vi "Get Available Operating Modes.vi"(8 "error in (no error)":errorcluster, 11 "VISA resource name":refnum<visa-resource-name>) -> (0 "error out":errorcluster, 2 "Operating Modes":i32[](array[ring]) items=["Weighing", "Parts Counting", "Deviations", "Dosing", "Formulas", "Animals Weighing", "Density", "Density of Solid Bodies", "Density of Liquids", "Peak Hold", "Totalizing", "Checkweighin", "Statistics", "Pipettes Calibration", "Differential Weighing", "Statistical Quality Control (SQC)", "Product Inspection", "Weight Control (Tableting)", "Drying", "Comparator", "Weighbridge"], 3 "VISA resource name out":refnum<visa-resource-name>)   [LabVIEW 2017, in "RadWag balances and scales.lvlib"]
doc: "Reads operating modes which are suported in connected balance.\nUsage of this VI is highly recommended before running VI \"Set Operating Mode\".\nTo see recommended usage of VI connected with seting operating mode open Examples ->RadWag Counting Pieces."
uses:
  <instrlib>/Prev/RadWag Continuous Read Folder/RadWag balances and scales.lvlib
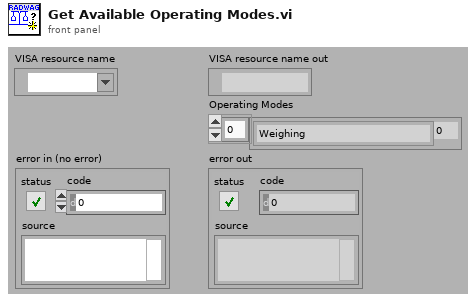
[diagram p1: front panel]
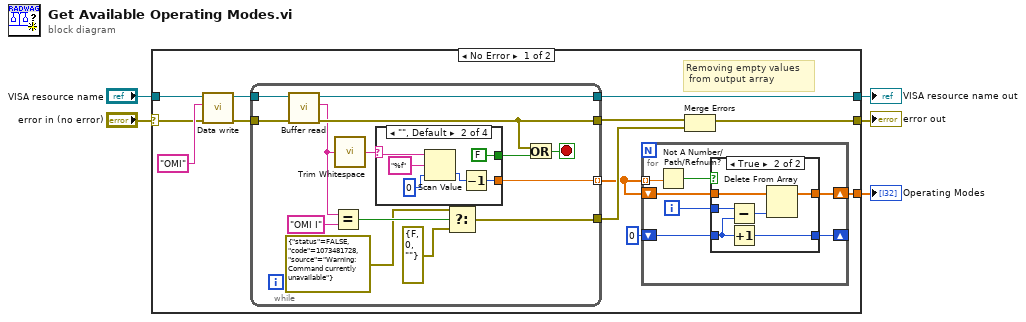
[diagram p0: block diagram]
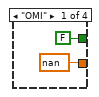
[diagram p3: hidden frame]
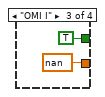
[diagram p4: hidden frame]
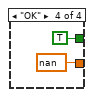
[diagram p5: hidden frame]
diagram:
  n1 = case shown="No Error" "error in (no error)" {
    selector: "error in (no error)" -> [w10 w59]
    tunnel: "VISA resource name" -> [w17 w60]
    tunnel: [w7 w59] -> w3
    tunnel: [w12 w60] -> w2
    tunnel: [w11 _] -> w1
    frame No Error {
      # "Removing empty values\n from output array"
      n2 = call <instrlib>:"Data write.vi"("error in (no error)"=w10, "ID"="OMI", "VISA resource name"=w17) -> ("error out"=w15:errorcluster, "VISA resource name out"=w16:refnum<visa-resource-name>)  [unwired: 7 in]
      n3 = while {
        tunnel: w16 -> [w46]
        tunnel: w15 -> [w45]
        tunnel: [w44] -> w12
        tunnel: [w42] -> w8
        tunnel: [w33] -> w6 mode=indexing
        tunnel: [w36] -> w9
        stop <- w40 stop-if-true
        n4 = call <instrlib>:"Buffer read.vi"("error in (no error)"=w45, "VISA resource name"=w46) -> ("error out"=w42:errorcluster, "Received String"=w35:string, "VISA resource name out"=w44:refnum<visa-resource-name>)  [unwired: 7 in]
        n5 = Equal?(x=w35, y="OMI I") -> (x = y?=w39:bool)
        n6 = call <vilib>:"Trim Whitespace.vi"("string"=w35) -> ("trimmed string"=w34:string)  [unwired: 1 in]
        n7 = case shown="\"\", Default" w34 {
          selector: w34 -> [_ w53 _ _]
          tunnel: [FALSE FALSE TRUE TRUE] -> w41
          tunnel: [nan w49 nan nan] -> w33
          frame "OMI" {
          }
          frame "", Default {
            n8 = Scan Value(string=w53, format string="%f", default (0 dbl)=0) -> (value=w50:i32)  [unwired: 1 out]
            n9 = Decrement(x=w50) -> (x-1=w49:i32)
          }
          frame "OMI I" {
          }
          frame "OK" {
          }
        }
        n10 = Select(t=errorcluster {"status"=FALSE, "code"=1073481728, "source"="Warning: Command currently unavailable"}, s=w39, f=errorcluster {"status"=FALSE, "code"=0, "source"=""} ("error constant")) -> (s? t:f=w36:errorcluster)
        n11 = Or(x=w42, y=w41) -> (x .or. y?=w40:bool)
      }
      n12 = for {
        tunnel: w6 -> [w22] mode=indexing
        shift-right: [w20] -> w11
        shift-left: w6 -> [w24]
        shift-right: [w18] -> _
        shift-left: 0 -> [w19]
        i -> [w23]
        n13 = Not A Number/Path/Refnum?(number/path/refnum=w22) -> (NaN/Path/Refnum?=w21:bool)
        n14 = case shown="True" w21 {
          tunnel: w24 -> [w26 w32]
          tunnel: w23 -> [_ w31]
          tunnel: [w26 w30] -> w20
          tunnel: w19 -> [w25 w27]
          tunnel: [w25 w29] -> w18
          frame False {
          }
          frame True {
            n15 = Subtract(x=w31, y=w27) -> (x-y=w28:i32)
            n16 = Increment(x=w27) -> (x+1=w29:i32)
            n17 = Delete From Array(array=w32, index=w28) -> (array with subset deleted=w30:dbl[])  [unwired: 1 in, 1 out]
          }
        }
      }
      n18 = Merge Errors(w8, w9) -> (w7:errorcluster)
    }
    frame Error {
    }
  }
  "error out" <- w3
  "VISA resource name out" <- w2
  "Operating Modes" <- w1
